vi "practiceMan.vi"() -> ()   [LabVIEW 2018]
uses:
  <vilib>/sound2/lvsound2.llb/Sound Data Format.ctl
  <vilib>/sound2/lvsound2.llb/Sampling Mode.ctl
  <vilib>/Utility/error.llb/DialogType.ctl
  <vilib>/sound2/lvsound2.llb/Sound File Info (path).vi
  <vilib>/sound2/lvsound2.llb/Sound File Read Open.vi
  <vilib>/sound2/lvsound2.llb/Sound File Read (DBL).vi
  <vilib>/measure/mascope.llb/Amplitude and Levels 1 chan.vi
  <vilib>/sound2/lvsound2.llb/Sound Output Write (DBL).vi
  <vilib>/measure/NI_MAPro.lvlib
panel:
  in  "Tab Control":enum32{"Normal use", "Debug page"}(tab)
  out "Prev. Session Active":bool
  in  "End Session":bool
  in  "Dev tab":bool
  out "Decibels":dbl(knob) scale=0.01..20.0 scale format="%#.10g"
  out "Amplifier Signal:":bool
  out "Silence":bool
  in  "Previous Session":bool
  out "data":waveform(dbl)[](graph)
  out "selected path":path
  in  "Device":u32
  in  "Play Waveform":bool
  in  "Pause Button":bool
  in  "Stop Button":bool
  in  "Restart Button":bool
  out "samples":i32
  out "Numeric":i32
  out "x-y":dbl
  out "total number of samples/ch":u32
  out "sound format":T1={"sample rate (S/s)"=22050.0, "number of channels"=2, "bits per sample"=16}
  out "error out 2":errorcluster
  out "error out 3":errorcluster
  out "error out":errorcluster
  out "error out 4":errorcluster
  out "Current Data":waveform(dbl)[](graph)
  # "Welcome to Practice, Man!\n\nClick \"Previous Session\" to begin"
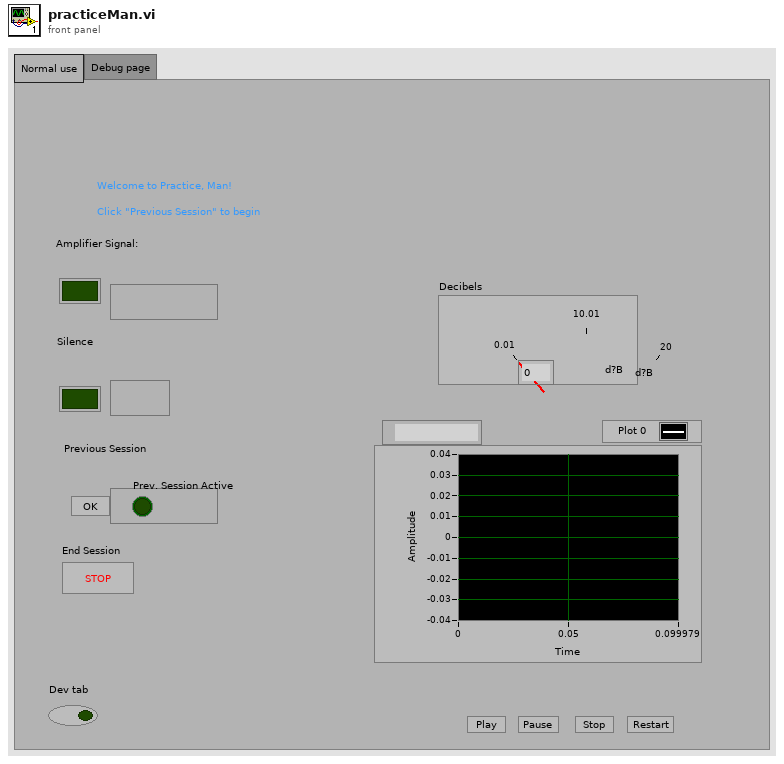
[diagram p1: front panel]
types:
  T1 = typedef "Sound Data Format.ctl" = cluster{"sample rate (S/s)":dbl, "number of channels":i32, "bits per sample":i32}
  T2 = typedef "Sampling Mode.ctl" = i32
  T3 = typedef "Sound Output Task ID.ctl" = u32
  T4 = typedef "Sound File Refnum.ctl" = refnum<file>
  T5 = typedef "DialogType.ctl" = u16
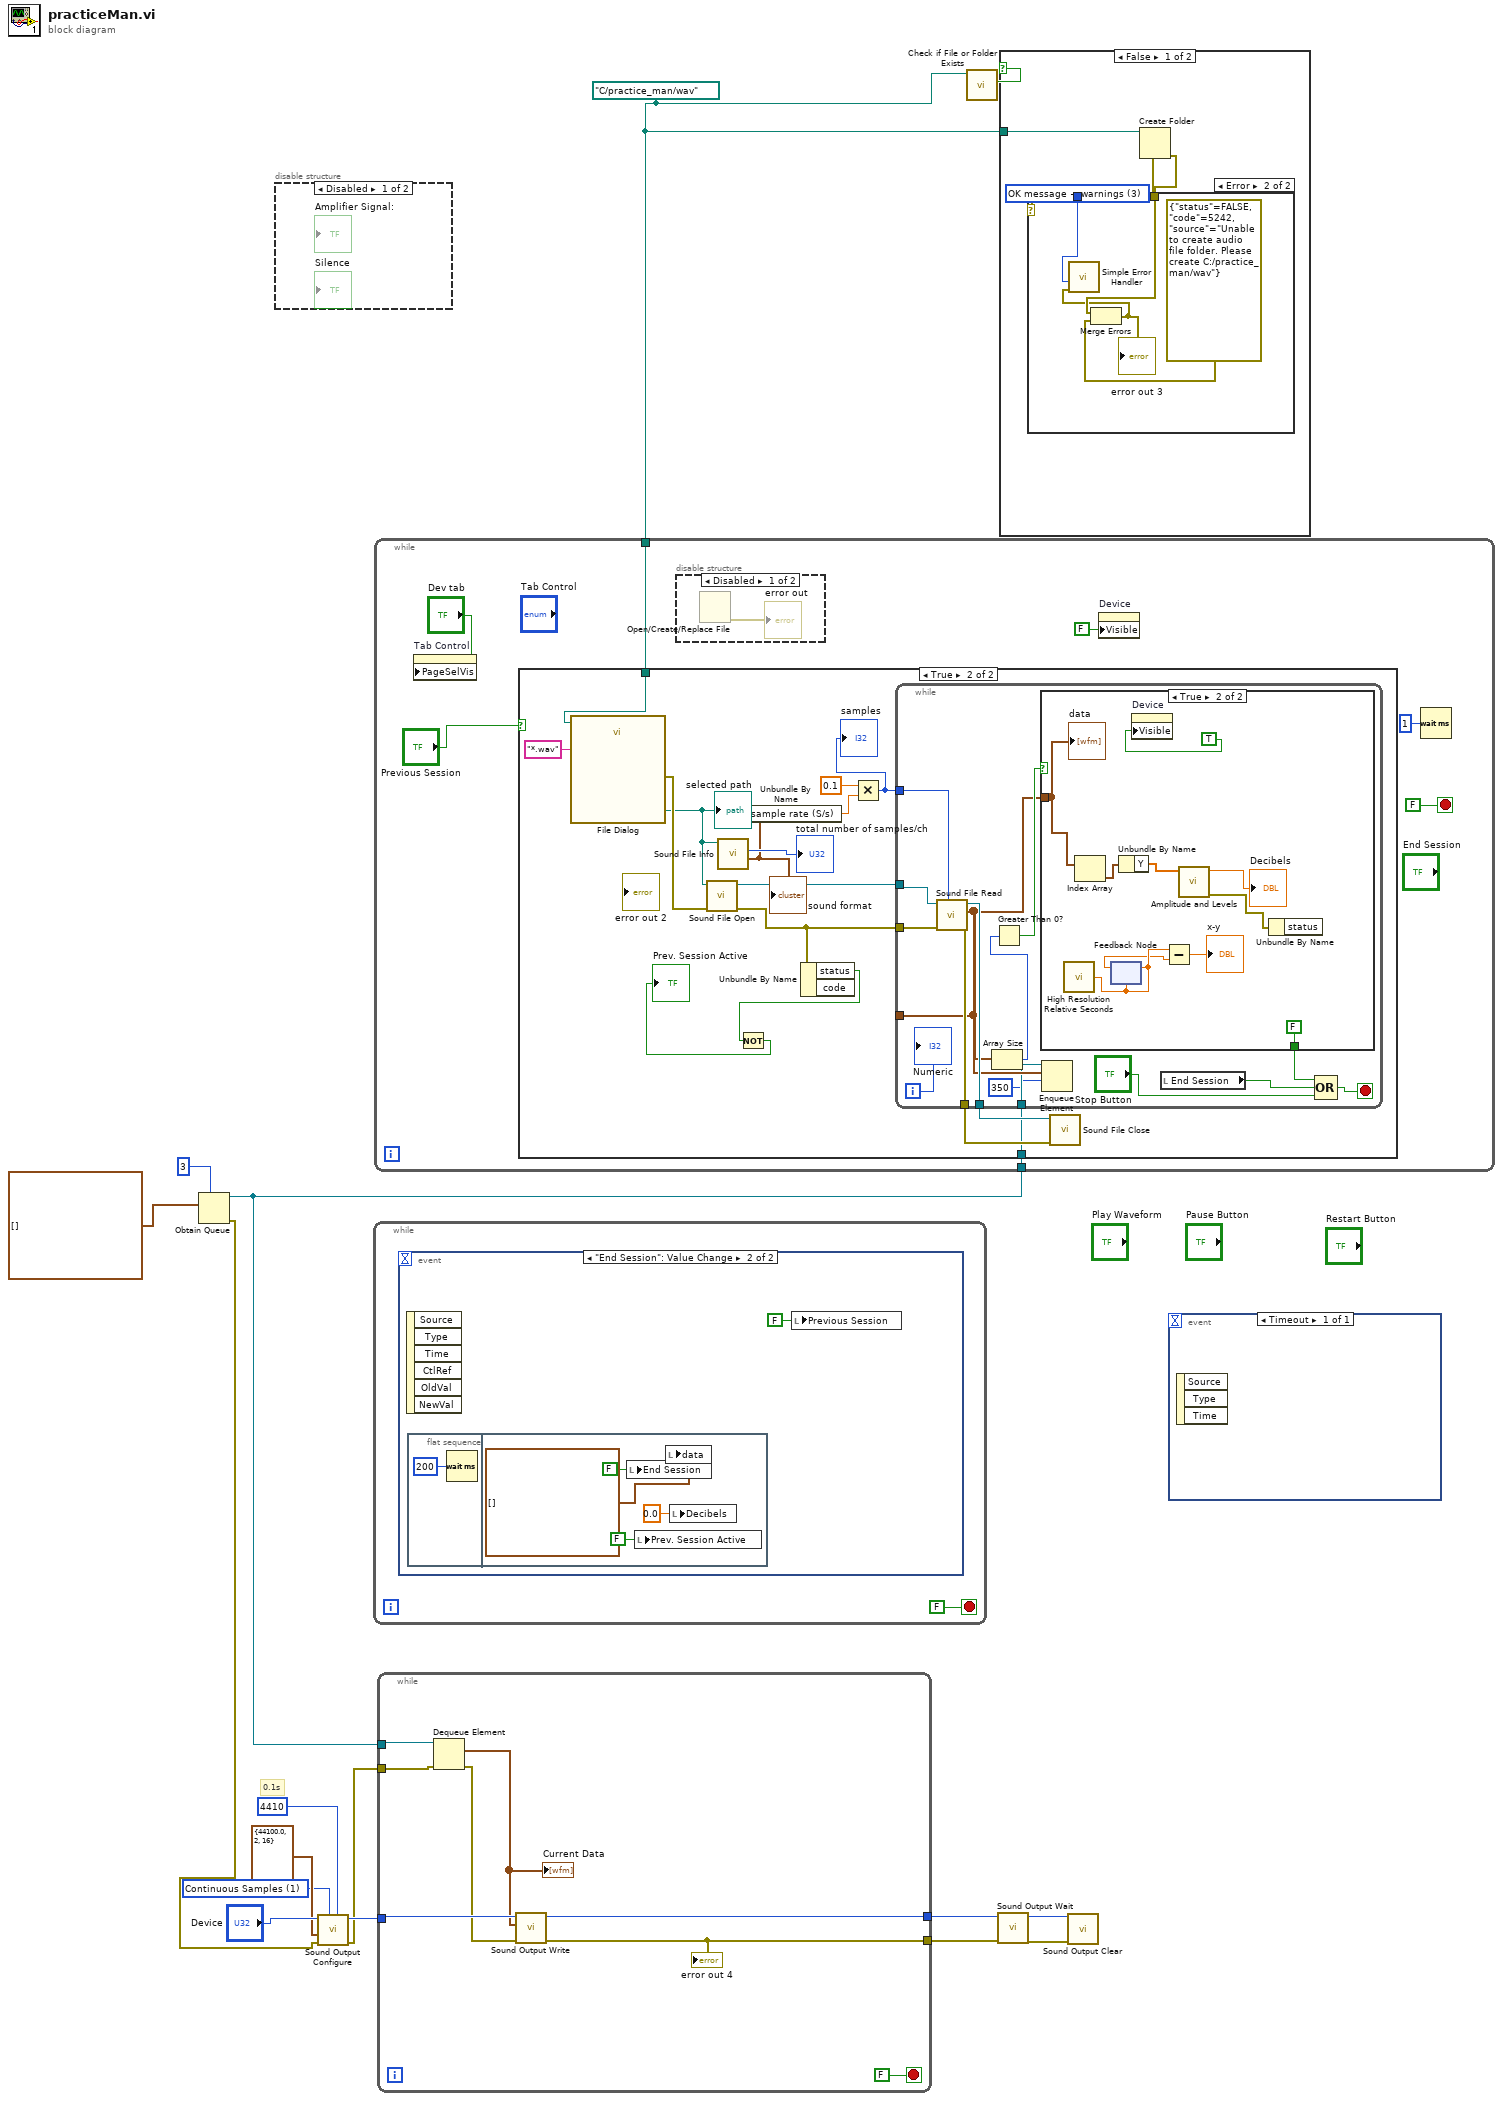
[diagram p0: block diagram]
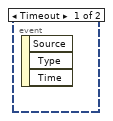
[diagram p2: hidden frame]
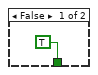
[diagram p8: hidden frame]
diagram:
  w8 = T2 1 items=["Finite Samples", "Continuous Samples"] ("sample mode")
  w15 = path "C:/practice_man/wav" ("start path")
  # "0.1s"
  n1 = Obtain Queue(max queue size (-1, unlimited)=3, element data type=waveform(dbl)[] [] ("data 2")) -> (queue out=w12:refnum<queue>, error out=w10:errorcluster)  [unwired: 3 in, 1 out]
  n2 = disable-structure shown="Disabled" {
    frame Disabled {
    }
    frame Enabled {
    }
  }
  n3 = call <vilib>:"Sound Output Configure.vi"("number of samples/ch"=4410, "sample mode"=w8, "error in (no error)"=w10, "sound format"=T1 {"sample rate (S/s)"=44100.0, "number of channels"=2, "bits per sample"=16} ("sound format 2"), "device ID"="Device") -> ("error out"=w5:errorcluster, "task ID"=w6:T3)  [unwired: 5 in]
  n4 = while {
    stop <- FALSE stop-if-true
    n5 = event shown="[1] \"End Session\": Value Change" {
      selector: _ -> [_ _]
      dyn-events: _ -> [_ _]
      timeout: _ -> [_ _]
      event Timeout {
        n6 = event-data() -> ()  [unwired: 1 in, 3 out]
      }
      event "End Session": Value Change {
        n7 = event-data() -> ()  [unwired: 1 in, 6 out]
        n8 = flat-sequence {
          frame #0 {
            n9 = Wait (ms)(milliseconds to wait=u32 200) -> ()  [unwired: 1 out]
          }
          frame #1 {
            n10 = local write "End Session"(FALSE ("End Session")) -> ()
            n11 = local write "Prev. Session Active"(FALSE ("Prev. Session Active")) -> ()
            n12 = local write "data"(waveform(dbl)[] [] ("data")) -> ()
            n13 = local write "Decibels"(0.0 ("Decibels")) -> ()
          }
        }
        n14 = local write "Previous Session"(FALSE ("Previous Session")) -> ()
      }
    }
  }
  n15 = while {
    tunnel: w15 -> [w28]
    tunnel: w12 -> [w24]
    stop <- FALSE stop-if-true
    n16 = property on="Tab Control" class="TabCtl (strict)"("PageSelVis"="Dev tab") -> ()  [unwired: 2 in, 2 out]
    n17 = case shown="True" "Previous Session" {
      tunnel: w28 -> [_ w47]
      tunnel: w24 -> [_ w32]
      frame False {
      }
      frame True {
        n18 = call "File Dialog"("start path"=w47, "pattern (all files)"="*.wav") -> ("selected path"=w44:path, "error out"=w46:errorcluster)  [unwired: 10 in, 2 out]
        "selected path" <- w44
        n19 = call-poly <vilib>:"Sound File Open.vi"("error in (no error)"=w46, "path"=w44) -> ("error out"=w35:errorcluster, "sound file refnum"=w45:T4)  [unwired: 8 in]
        n20 = call-poly <vilib>:"Sound File Info.vi"("path"=w44) -> ("sound format"=w37:T1, "total number of samples/ch"=→"total number of samples/ch":u32)  [unwired: 7 in, 2 out]
        "sound format" <- w37
        n21 = Unbundle By Name(w37) -> ("sample rate (S/s)"=w36:dbl)
        n22 = Unbundle By Name(w35) -> ("status"=w34:bool)  [unwired: 1 out]
        n23 = Not(x=w34) -> (.not. x?=→"Prev. Session Active":bool)
        n24 = Multiply(x=0.1, y=w36) -> (x*y=w38:i32)
        "samples" <- w38
        n25 = while {
          tunnel: w45 -> [w62]
          tunnel: w35 -> [w61]
          tunnel: [w58] -> w43
          tunnel: [w57] -> w42
          tunnel: w38 -> [w56]
          tunnel: w32 -> [w49]
          tunnel: [w50] -> _
          i -> [w55]
          stop <- w52 stop-if-true
          n26 = call-poly <vilib>:"Sound File Read.vi"("number of samples/ch (-1: all)"=w56, "error in (no error)"=w61, "sound file refnum"=w62) -> ("error out"=w58:errorcluster, "data"=w50:waveform(dbl)[], "sound file refnum out"=w57:T4)  [unwired: 4 in, 2 out]
          n27 = Array Size(array=w50) -> (size(s)=w60:i32)
          n28 = Greater Than 0?(x=w60) -> (x > 0?=w59:bool)
          n29 = case shown="True" w59 {
            tunnel: w50 -> [_ w64]
            tunnel: [TRUE FALSE] -> w54
            frame False {
            }
            frame True {
              n30 = call <vilib>:"High Resolution Relative Seconds.vi"() -> ("relative seconds"=w67:dbl)
              n31 = Index Array(array=w64) -> (element=w71:waveform(dbl))  [unwired: 1 in]
              n32 = feedback-in #1(w67) -> ()
              n33 = feedback #1(w67) -> (w66:dbl)
              n34 = Unbundle By Name(w71) -> ("Y"=w70:dbl[])
              n35 = property on="Device" class="DigNum (strict)"("Visible"=TRUE) -> ()  [unwired: 2 in, 2 out]
              n36 = Subtract(x=w67, y=w66) -> (x-y=→"x-y":dbl)
              n37 = call-poly <vilib>:"Amplitude and Levels.vi"("signal in"=w70) -> ("error out"=w65:errorcluster, "amplitude"=→"Decibels":dbl)  [unwired: 7 in, 2 out]
              n38 = Unbundle By Name(w65) -> ()  [unwired: 1 out]
              "data" <- w64
            }
          }
          n39 = Enqueue Element(queue=w49, element=w50, timeout in ms (-1)=350) -> ()  [unwired: 1 in, 3 out]
          n40 = local read "End Session"() -> (w53:bool)
          n41 = Compound Arithmetic op=OR(w54, w53, "Stop Button") -> (w52:bool)
          "Numeric" <- w55
        }
        n42 = call <vilib>:"Sound File Close.vi"("error in (no error)"=w43, "sound file refnum"=w42) -> ()  [unwired: 9 in, 1 out]
      }
    }
    n43 = disable-structure shown="Disabled" {
      frame Disabled {
        n44 = Open/Create/Replace File() -> (error out=→"error out":errorcluster)  [unwired: 6 in, 2 out]
      }
      frame Enabled {
      }
    }
    n45 = property on="Device" class="DigNum (strict)"("Visible"=FALSE) -> ()  [unwired: 2 in, 2 out]
    n46 = Wait (ms)(milliseconds to wait=u32 1) -> ()  [unwired: 1 out]
  }
  n47 = while {
    tunnel: w12 -> [w81]
    tunnel: w6 -> [w78]
    tunnel: w5 -> [w79]
    tunnel: [w76] -> w4
    tunnel: [w75] -> w3
    stop <- FALSE stop-if-true
    n48 = Dequeue Element(queue=w81, error in (no error)=w79) -> (element=w74:waveform(dbl)[], error out=w77:errorcluster)  [unwired: 1 in, 2 out]
    "Current Data" <- w74
    n49 = call-poly <vilib>:"Sound Output Write.vi"("error in (no error)"=w77, "data"=w74, "task ID"=w78) -> ("error out"=w75:errorcluster, "task ID out"=w76:T3)  [unwired: 7 in]
    "error out 4" <- w75
  }
  n50 = call <vilib>:"Check if File or Folder Exists.vi"("path"=w15) -> ("file or folder exists?"=w16:bool)  [unwired: 8 in, 2 out]
  n51 = call <vilib>:"Sound Output Wait.vi"("error in (no error)"=w3, "task ID"=w4) -> ("error out"=w2:errorcluster, "task ID out"=w1:T3)  [unwired: 8 in]
  n52 = case shown="False" w16 {
    tunnel: w15 -> [w84 _]
    frame False {
      w83 = T5 3 items=["no dialog", "OK message", "continue or stop message", "OK message + warnings", "continue/stop + warnings"] ("type of dialog (OK msg:1)")
      n53 = Create Folder(path (use dialog)=w84) -> (error out=w82:errorcluster)  [unwired: 2 in, 2 out]
      n54 = case shown="Error" w82 {
        tunnel: w83 -> [_ w88]
        tunnel: w82 -> [_ w87]
        frame No Error {
        }
        frame Error {
          n55 = Merge Errors(w87, errorcluster {"status"=FALSE, "code"=5242, "source"="Unable to create audio file folder. Please create C:/practice_man/wav"} ("error out 3")) -> (w85:errorcluster)
          "error out 3" <- w85
          n56 = call <vilib>:"Simple Error Handler.vi"("type of dialog (OK msg:1)"=w88, "error in (no error)"=w85) -> ()  [unwired: 3 in, 5 out]
        }
      }
    }
    frame True {
    }
  }
  n57 = call <vilib>:"Sound Output Clear.vi"("error in (no error)"=w2, "task ID"=w1) -> ()  [unwired: 9 in, 1 out]
  n58 = event shown="[0] Timeout" {
    selector: _ -> [_]
    dyn-events: _ -> [_]
    timeout: _ -> [_]
    event Timeout {
      n59 = event-data() -> ()  [unwired: 1 in, 3 out]
    }
  }
